vi "remove(byVal).vi"(6 "Remove Dependencies?":bool, 10 "UniqueName in":refnum<class "UniqueName.lvclass">, 11 "NameRegistry in":refnum<class "NameRegistry.lvclass">) -> (1 "Dependencies removed":string[](array[string]), 2 "Fully Qualified Name":string, 3 "NameRegistry out":refnum<class "NameRegistry.lvclass">)   [LabVIEW 2013, in "UniqueName.lvlib" / "NameRegistry.lvclass"]
uses:
  NameRegistry.lvclass
  UniqueNameClass/UniqueName.lvclass
  <vilib>/regexp/Match Regular Expression.xnode
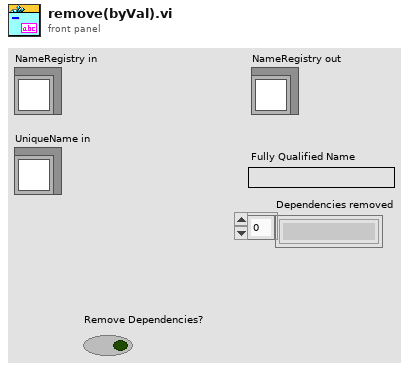
[diagram p1: front panel]
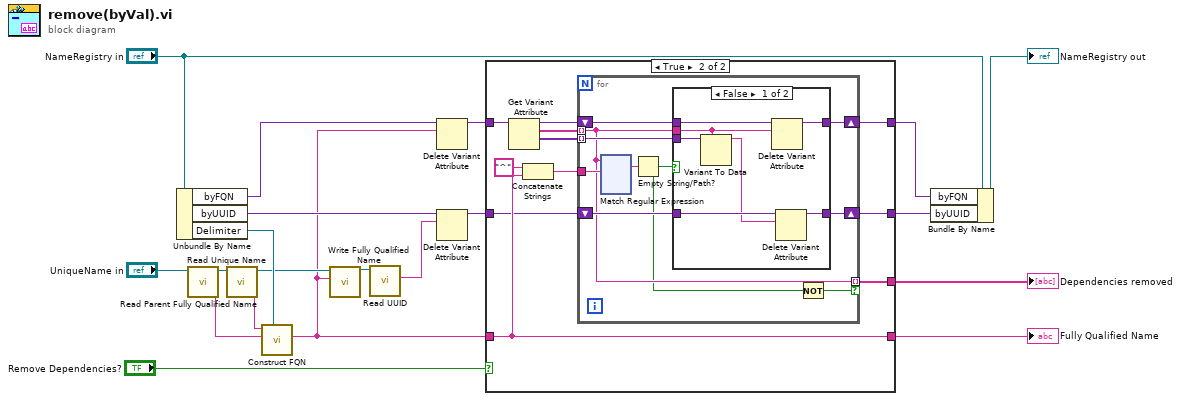
[diagram p0: block diagram]
diagram:
  n1 = Unbundle By Name("NameRegistry in") -> ("byFQN"=w18:variant, "byUUID"=w20:variant, "Delimiter"=w16:refnum<class "Delimiter.lvclass">)
  n2 = call "Read Unique Name.vi"("UniqueName in"="UniqueName in") -> ("Unique Name"=w14:string, "UniqueName out"=w13:refnum<class "UniqueName.lvclass">)  [unwired: 9 in]
  n3 = call "Read Parent Fully Qualified Name.vi"("UniqueName in"=w13) -> ("Parent Fully Qualified Name"=w11:string, "UniqueName out"=w12:refnum<class "UniqueName.lvclass">)  [unwired: 9 in]
  n4 = call "Construct FQN.vi"("Delimiter"=w16, "Name"=w14, "Parent FQN"=w11) -> ("FQN"=w2:string)  [unwired: 8 in]
  n5 = call "Write Fully Qualified Name.vi"("Fully Qualified Name"=w2, "UniqueName in"=w12) -> ("UniqueName out"=w19:refnum<class "UniqueName.lvclass">)  [unwired: 9 in]
  n6 = call "Read UUID.vi"("UniqueName in"=w19) -> ("UUID"=w9:string)  [unwired: 9 in, 1 out]
  n7 = Delete Variant Attribute(6:w2, 7:w18) -> (3:w7:variant)  [unwired: 1 in, 2 out]
  n8 = Delete Variant Attribute(6:w9, 7:w20) -> (3:w5:variant)  [unwired: 1 in, 2 out]
  n9 = case shown="True" "Remove Dependencies?" {
    tunnel: w7 -> [w23 w34]
    tunnel: [w23 w28] -> w6
    tunnel: w5 -> [w22 w26]
    tunnel: [w22 w27] -> w4
    tunnel: [w21 w32] -> w3
    tunnel: w2 -> [w21 w32]
    tunnel: [_ w24] -> w1
    frame False {
    }
    frame True {
      n10 = Get Variant Attribute(Variant=w34) -> (duplicate Variant=w29:variant, names=w33:string[], values=w25:variant[])  [unwired: 3 in, 1 out]
      n11 = Concatenate Strings("^" ("string"), w32) -> (w30:string)
      n12 = for {
        tunnel: w33 -> [w37] mode=indexing
        tunnel: w30 -> [w44]
        shift-right: [w41] -> w28
        shift-left: w29 -> [w42]
        shift-right: [w40] -> w27
        shift-left: w26 -> [w39]
        tunnel: w25 -> [w38] mode=indexing
        tunnel: [w37] -> w24 mode=indexing if=w35
        n13 = xnode "Match Regular Expression"("input string"=w37, "regular expression"=w44) -> ("whole match"=w43:string)  [unwired: 4 in, 4 out]
        n14 = Empty String/Path?(string/path=w43) -> (empty?=w36:bool)
        n15 = case shown="False" w36 {
          tunnel: w42 -> [w51 w53]
          tunnel: [w50 w53] -> w41
          tunnel: [w47 w52] -> w40
          tunnel: w39 -> [w46 w52]
          tunnel: w38 -> [w49 _]
          tunnel: w37 -> [w48 _]
          frame False {
            n16 = Variant To Data(type=w48, Variant=w49) -> (data=w45:string)  [unwired: 1 in, 1 out]
            n17 = Delete Variant Attribute(6:w48, 7:w51) -> (3:w50:variant)  [unwired: 1 in, 2 out]
            n18 = Delete Variant Attribute(6:w45, 7:w46) -> (3:w47:variant)  [unwired: 1 in, 2 out]
          }
          frame True {
          }
        }
        n19 = Not(x=w36) -> (.not. x?=w35:bool)
      }
    }
  }
  "Fully Qualified Name" <- w3
  "Dependencies removed" <- w1
  n20 = Bundle By Name(cluster="NameRegistry in", "byFQN"=w6, "byUUID"=w4) -> (→"NameRegistry out":refnum<class "NameRegistry.lvclass">)
